vi "Remote Panels Globals.vi"() -> ()   [LabVIEW 2017]
panel:
  out "Stop Server":bool
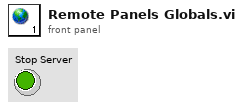
[diagram p1: front panel]
diagram:
